vi "Test Snake Move Horizontally Outside World.vi"(8 "error in (no error)":errorcluster, 11 "Test Case In":refnum<class "World Test.lvclass">) -> (0 "error out":errorcluster, 3 "Test Case Out":refnum<class "World Test.lvclass">)   [LabVIEW 2020, in "World Test.lvclass"]
uses:
  World Test.lvclass
  C:/Program Files (x86)/National Instruments/LabVIEW 2020/vi.lib/Astemes/LUnit/Test Case.lvclass
  source/Particle/Position.ctl
  source/Snake/Direction.ctl
  <vilib>/Astemes/LUnit/Test Case.lvclass/Test Case.ctl
  <vilib>/Astemes/LUnit/Palette/Fail.vi
  <vilib>/Astemes/LUnit/Palette/Pass.vi
  <vilib>/Astemes/LUnit/Set Assertion Type.vi
  <vilib>/Astemes/LUnit/Add test result.vi
  <vilib>/Astemes/LUnit/LUnit Record Assertion Result.vi
  <vilib>/Astemes/LUnit/LUnit Aggregate Assertion Results.vi
  <vilib>/Astemes/LUnit/Method Result/LUnit Merge Status.vi
  <vilib>/Astemes/LUnit/LUnit Concatenate result strings.vi
  source/World/World.lvclass
  source/Particle.lvclass
  source/Snake/Snake.lvclass
  <vilib>/Astemes/LUnit/Test Case.lvclass
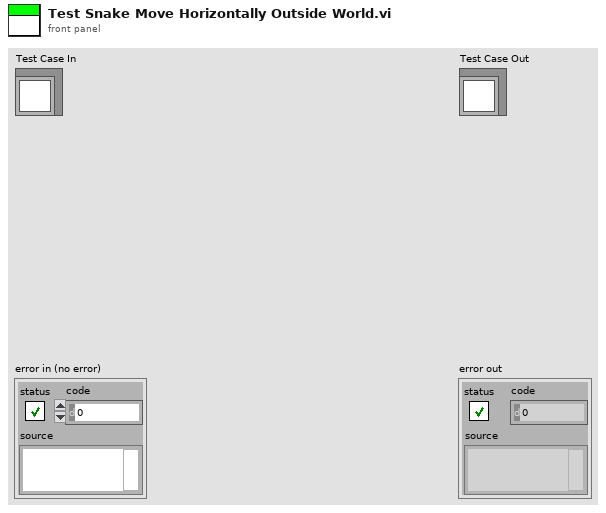
[diagram p1: front panel]
types:
  T1 = typedef "Snake.lvclass/Direction.ctl" = enum16{"X", "-X", "Y", "-Y"}
  T2 = typedef "Particle.lvclass/Position.ctl" = cluster{"X":i32, "Y":i32}
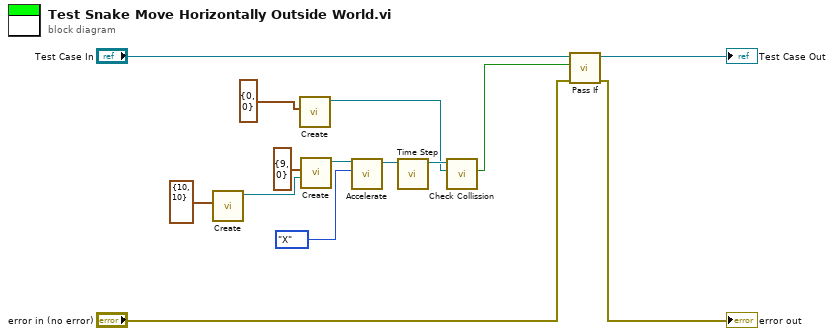
[diagram p0: block diagram]
diagram:
  n1 = call "Create.vi"("Size"=T2 {"X"=10, "Y"=10}) -> ("World out"=w9:refnum<class "World.lvclass">)  [unwired: 10 in]
  n2 = call "Create.vi"("Position"=T2 {"X"=0, "Y"=0}) -> ("Particle out"=w3:refnum<class "Particle.lvclass">)  [unwired: 10 in]
  n3 = call "Create.vi"("World.lvclass"=w9, "Position"=T2 {"X"=9, "Y"=0}) -> ("Snake out"=w7:refnum<class "Snake.lvclass">)  [unwired: 9 in]
  n4 = call "Accelerate.vi"("Direction"=Direction."X", "Snake in"=w7) -> ("Snake out"=w6:refnum<class "Snake.lvclass">)  [unwired: 9 in]
  n5 = call "Time Step.vi"("Snake in"=w6) -> ("Snake out"=w4:refnum<class "Snake.lvclass">)  [unwired: 10 in]
  n6 = call "Check Collission.vi"("Particle"=w3, "Snake in"=w4) -> ("Collided?"=w2:bool)  [unwired: 8 in, 1 out]
  n7 = call <vilib>:"Pass If.vi"("error in (no error)"="error in (no error)", "Pass?"=w2, "LUnit Test Case In"="Test Case In") -> ("error out"=→"error out":errorcluster, "LUnit Test Case Out"=→"Test Case Out":refnum<class "World Test.lvclass">)  [unwired: 7 in]
